vi "testV3-SensorReadtimeWritefile.vi"() -> ()   [LabVIEW 2020]
uses:
  <vilib>/DAQmx/read.llb/DAQmx Read (Analog 2D DBL NChan NSamp).vi
  <vilib>/Analysis/baseanly.llb/Mean (DBL).vi
  <vilib>/DAQmx/miscellaneous.llb/DAQmx Fill In Error Info.vi
  <vilib>/Analysis/NI_AALBase.lvlib
  <resource>/objmgr/daqmx.rc
panel:
  out "transposed array":dbl[][](array[numeric])
  out "size(s)":i32
  out "x/y":dbl
  in  "Sampling Time":u32
  in  "DAQmx Task Name 2":refnum<k21>
  in  "Read Time (s) 2":u32
  out "Array":dbl[][](array[numeric])
  in  "stop":bool
  out "F-format string":string[](array[string])
  in  "Path":path
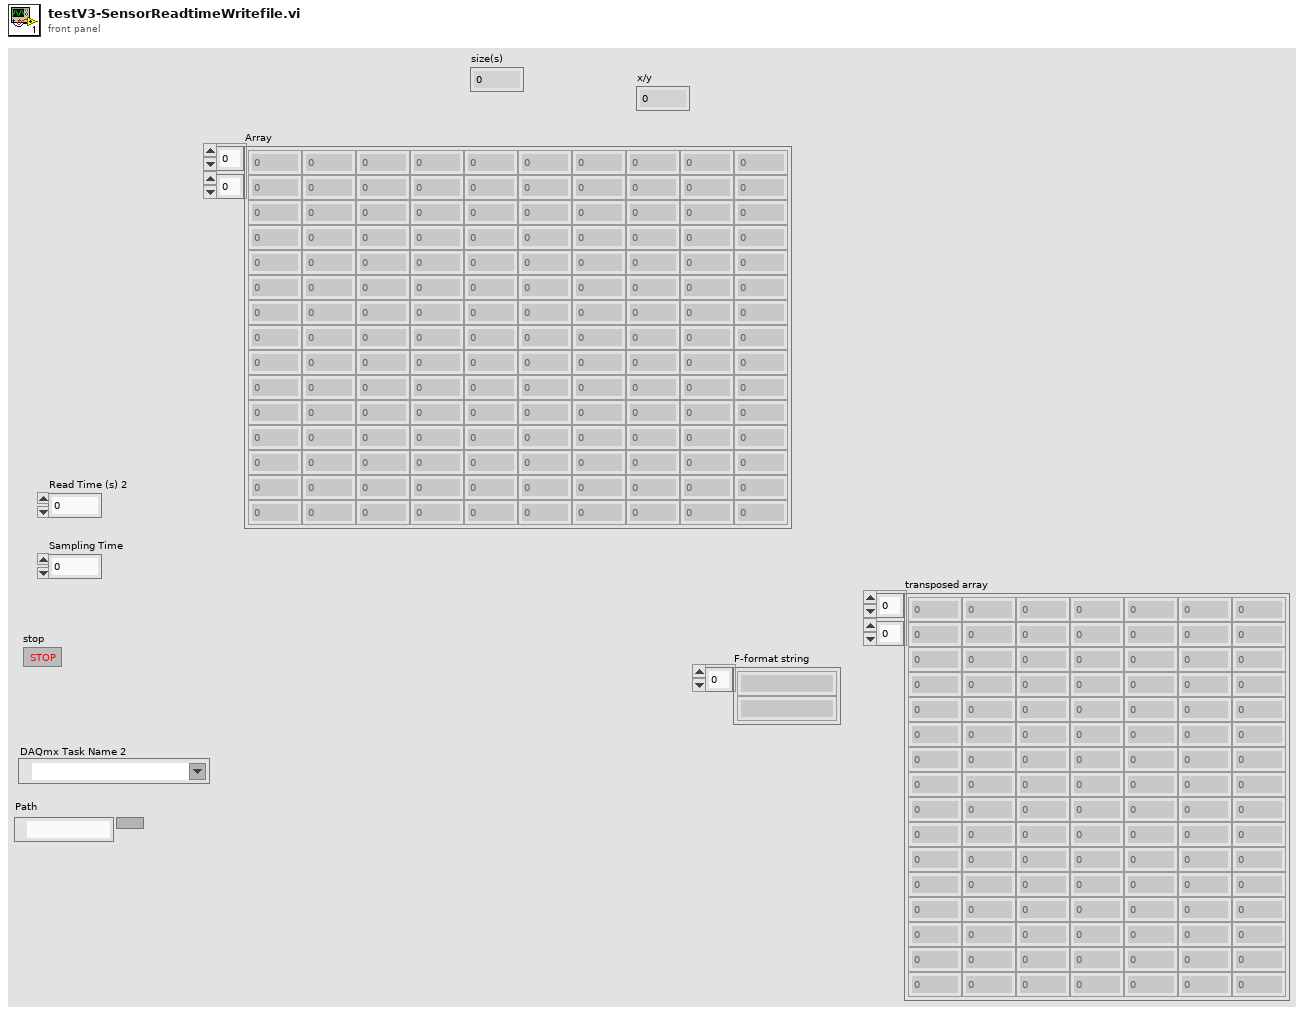
[diagram p1: front panel]
types:
  T1 = enum16{"open", "replace", "create", "open or create", "replace or create", "replace or create with confirmation"}
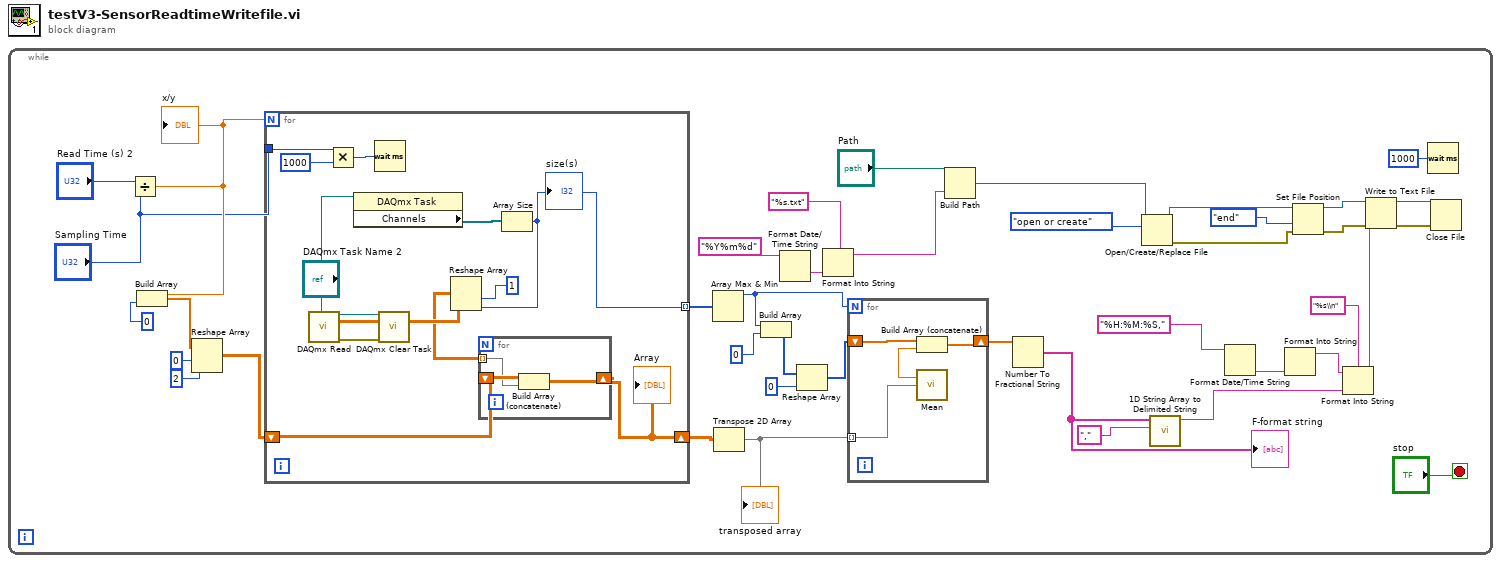
[diagram p0: block diagram]
diagram:
  n1 = while {
    stop <- "stop" stop-if-true
    n2 = Divide(x="Read Time (s) 2", y="Sampling Time") -> (x/y=w10:dbl)
    "x/y" <- w10
    n3 = Build Array(w10, 0 ("element")) -> (w15:dbl[])
    n4 = Reshape Array(w15, 0 ("dimension size"), 2 ("dimension size")) -> (w12:dbl[][])
    n5 = for {
      N: w10 -> [_]
      shift-right: [w49] -> w7
      shift-left: w12 -> [w48]
      tunnel: "Sampling Time" -> [w47]
      tunnel: [w42] -> w8 mode=indexing
      n6 = call-poly <vilib>:"DAQmx Read.vi"("task/channels in"="DAQmx Task Name 2") -> ("task out"=w53:refnum<k21>, "data"=w51:dbl[][], "error out"=w54:errorcluster)  [unwired: 12 in]
      n7 = Multiply(x=w47, y=u32 1000) -> (x*y=w45:u32)
      n8 = property class="DAQmx Task"(reference="DAQmx Task Name 2") -> ("Channels"=w44:refnum<k21>[])  [unwired: 1 in, 2 out]
      n9 = Wait (ms)(milliseconds to wait=w45) -> ()  [unwired: 1 out]
      n10 = call <vilib>:"DAQmx Clear Task.vi"("task in"=w53, "error in"=w54) -> ()  [unwired: 13 in, 1 out]
      n11 = Array Size(array=w44) -> (size(s)=w42:i32)
      "size(s)" <- w42
      n12 = Reshape Array(w51, 1 ("dimension size"), w42) -> (w50:dbl[][])
      n13 = for {
        shift-right: [w56] -> w49
        shift-left: w48 -> [w57]
        tunnel: w50 -> [w55] mode=indexing
        n14 = Build Array (concatenate)(w57, w55) -> (w56:dbl[][])
      }
      "Array" <- w49
    }
    n15 = Array Max & Min(array=w8) -> (max value=w4:i32)  [unwired: 3 out]
    n16 = Transpose 2D Array(2D array=w7) -> (transposed array=w6:dbl[][])
    "transposed array" <- w6
    n17 = Build Array(w4, 0 ("element")) -> (w2:i32[])
    n18 = Format Date/Time String(time format string (%c)="%Y%m%d") -> (date/time string=w28:string)  [unwired: 2 in]
    n19 = Reshape Array(w2, 0 ("dimension size")) -> (w1:i32[])
    n20 = Format Into String(format string="%s.txt", w28) -> (resulting string=w25:string)  [unwired: 2 in, 1 out]
    n21 = for {
      N: w4 -> [_]
      tunnel: w6 -> [w61] mode=indexing
      shift-right: [w59] -> w17
      shift-left: w1 -> [w58]
      n22 = call-poly <vilib>:"Mean.vi"("X"=w61) -> ("mean"=w60:dbl)  [unwired: 1 out]
      n23 = Build Array (concatenate)(w58, w60) -> (w59:dbl[])
    }
    n24 = Build Path(base path="Path", name or relative path=w25) -> (appended path=w24:path)
    n25 = Number To Fractional String(number=w17) -> (F-format string=w18:string[])  [unwired: 3 in]
    "F-format string" <- w18
    n26 = Open/Create/Replace File(file path (use dialog)=w24, operation (0:open)=T1."open or create") -> (refnum out=w37:refnum<file>, error out=w34:errorcluster)  [unwired: 4 in, 1 out]
    n27 = call <vilib>:"1D String Array to Delimited String.vi"("delimiter"="," ("format string"), "string array"=w18) -> ("delimited string"=w23:string)  [unwired: 9 in]
    n28 = Format Date/Time String(time format string (%c)="%H:%M:%S,") -> (date/time string=w20:string)  [unwired: 2 in]
    n29 = Format Into String(w20) -> (resulting string=w19:string)  [unwired: 3 in, 1 out]
    n30 = Set File Position(refnum=w37, from (0:start)=enum16{"start", "end", "current"}."end", error in=w34) -> (refnum out=w36:refnum<file>, error out=w33:errorcluster)  [unwired: 1 in]
    n31 = Format Into String(format string="%s\\n", initial string=w19, w23) -> (resulting string=w30:string)  [unwired: 1 in, 1 out]
    n32 = Write to Text File(file (use dialog)=w36, text=w30, error in=w33) -> (refnum out=w35:refnum<file>, error out=w32:errorcluster)  [unwired: 1 in, 1 out]
    n33 = Wait (ms)(milliseconds to wait=u32 1000) -> ()  [unwired: 1 out]
    n34 = Close File(refnum=w35, error in=w32) -> ()  [unwired: 2 out]
  }
